vi "Modus zu String.vi"(11 "Modus":T1 caption="Modus:" items=["CG zu PNS", "CG zu Entnahmestelle"]) -> (3 "Modus String":string)   [LabVIEW 2020, in "Linearisierung v2.lvlib" / "SpanEinstellungen.lvlib"]
uses:
  SpanEinstellungen.lvlib
  EPA 1065/T90 1065-308/Modus.ctl
  EPA 1065/T90 1065-308/T90 Test 1065-308.lvlib
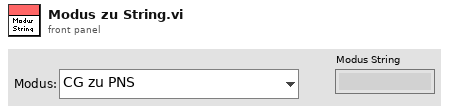
[diagram p1: front panel]
types:
  T1 = typedef "EPA 1065.lvlib/T90 Test 1065-308.lvlib/Modus.ctl" = u16
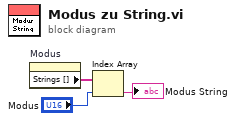
[diagram p0: block diagram]
diagram:
  n1 = property on="Modus" class="Ring (strikt)"() -> ("Strings []"=w3:string[])  [unwired: 2 in, 2 out]
  n2 = Index Array(array=w3, index="Modus") -> (element=→"Modus String":string)
